vi "THzTimeScan_830_VC.vi"(0 "input":T1) -> (1 "loop stop":bool, 2 "x-axis":sgl[](array[numeric]), 3 "y-axis":dbl[](array[numeric]))   [LabVIEW 2010]
uses:
  <vilib>/Utility/file.llb/Write To Spreadsheet File (string).vi
panel:
  out "Position":dbl[](array[numeric])=[3.9963] format="%.6f"
  out "Array":dbl[](array[numeric])
  out "String":string
  out "Move delay":bool
  out "Read830":bool
  out "THz Signal Graph":dbl(graph)
  in  "loop stop":bool
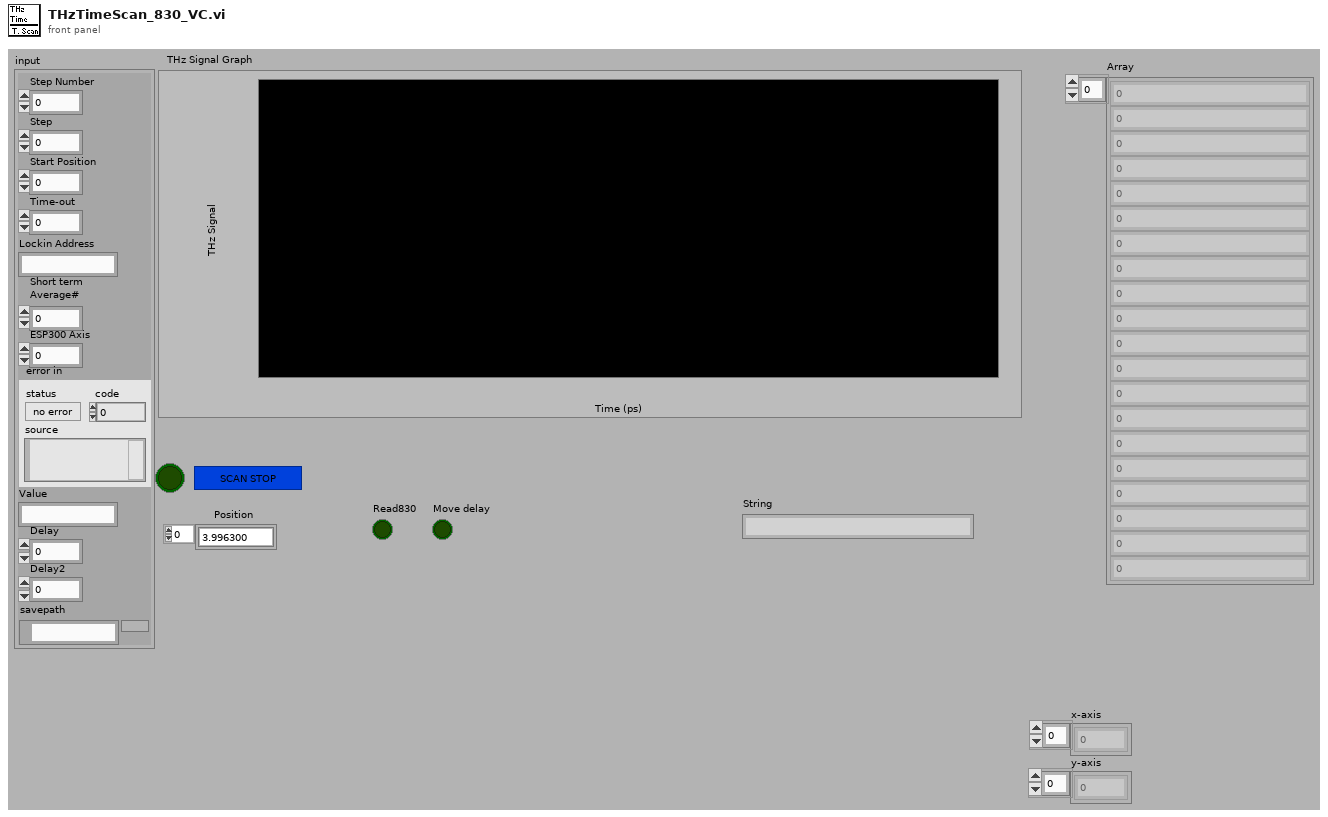
[diagram p1: front panel]
types:
  T1 = cluster{"Step Number":i32, "Step":sgl, "Start Position":sgl, "Time-out":i32, "Lockin Address":string, "Short term \nAverage#":i8, "ESP300 Axis":i8, "error in":errorcluster, "Value":string, "Delay":dbl, "Delay2":dbl, "savepath":path}
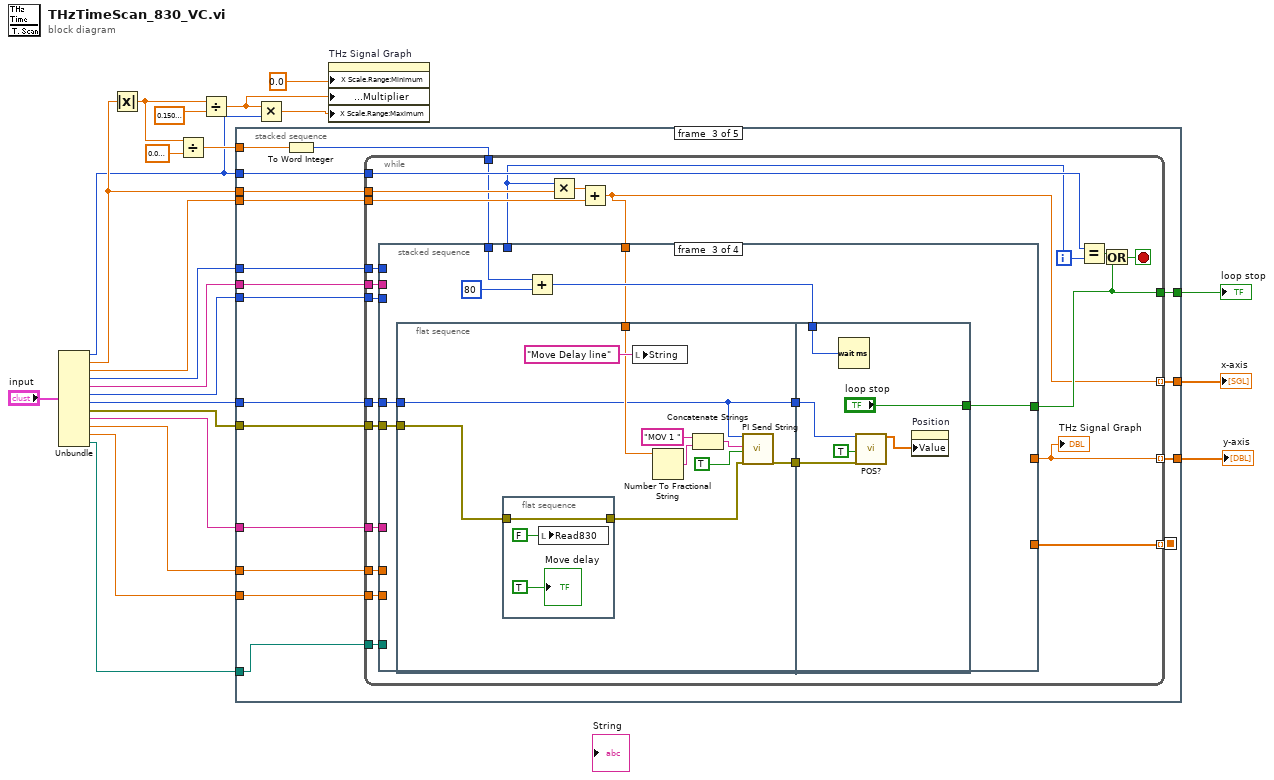
[diagram p0: block diagram]
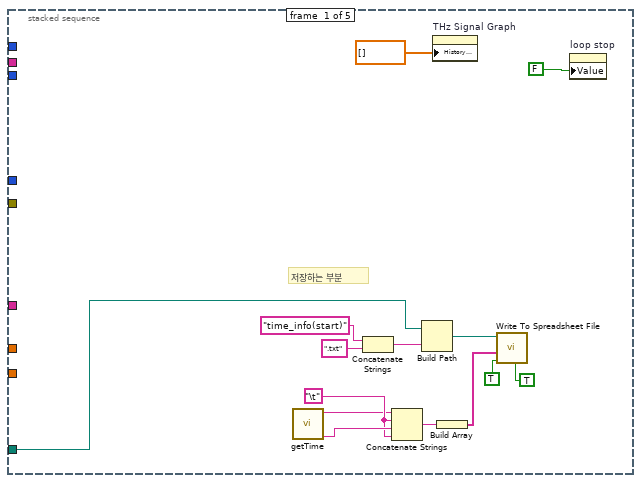
[diagram p2: hidden frame]
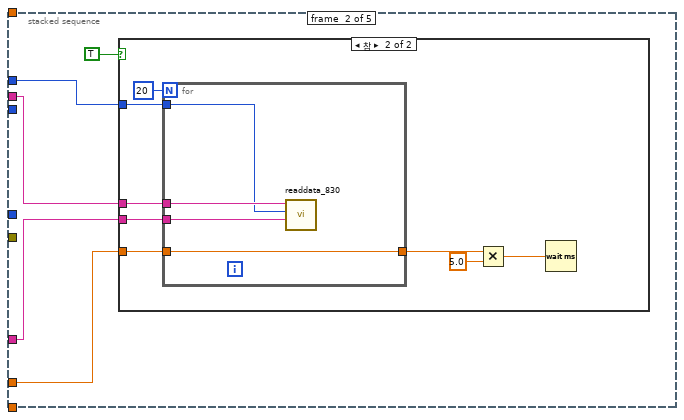
[diagram p3: hidden frame]
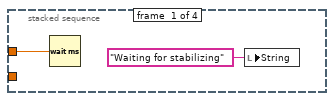
[diagram p5: hidden frame]
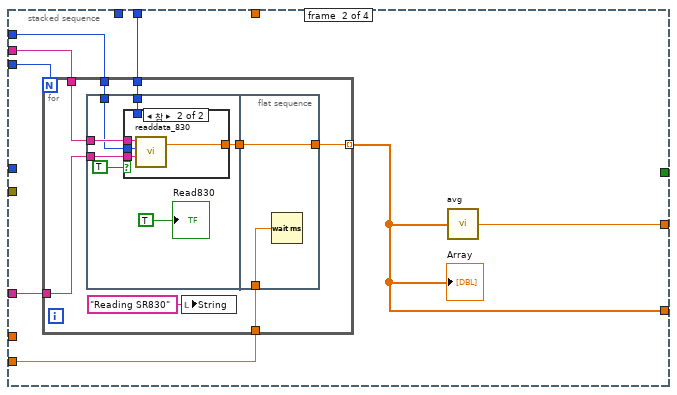
[diagram p6: hidden frame]
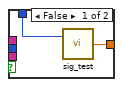
[diagram p7: hidden frame]
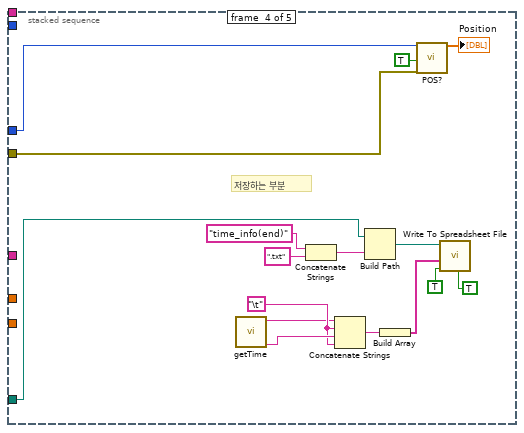
[diagram p9: hidden frame]
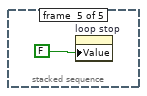
[diagram p10: hidden frame]
diagram:
  n1 = Unbundle("input") -> ("Step Number"=w9:i32, "Step"=w15:sgl, "Start Position"=w14:sgl, "Time-out"=w13:i32, "Lockin Address"=w12:string, "Short term \nAverage#"=w5:i8, "ESP300 Axis"=w11:i8, "error in"=w1:errorcluster, "Value"=w10:string, "Delay"=w4:dbl, "Delay2"=w3:dbl, "savepath"=w2:path)
  n2 = Absolute Value(x=w15) -> (abs(x)=w19:sgl)
  n3 = Divide(x=w19, y=sgl 0.004) -> (x/y=w17:sgl)
  n4 = Divide(x=w19, y=sgl 0.15) -> (x/y=w7:sgl)
  n5 = stacked-sequence {
    seq-local: [_ _ w58 _ _] -> [_ _ _ _ _]
    tunnel: w14 -> [_ _ w72 _ _]
    tunnel: w13 -> [_ w42 w71 _ _]
    tunnel: w12 -> [_ w41 w70 _ _]
    tunnel: w5 -> [_ _ w69 _ _]
    tunnel: w11 -> [_ _ w56 w156 _]
    tunnel: w1 -> [_ _ w55 w155 _]
    tunnel: w10 -> [_ w40 w61 _ _]
    tunnel: [_ _ w68 _ _] -> w23
    tunnel: [_ _ w67 _ _] -> w22
    tunnel: [_ _ w66 _ _] -> w21
    tunnel: w15 -> [_ _ w64 _ _]
    tunnel: w9 -> [_ _ w65 _ _]
    tunnel: w17 -> [_ _ w63 _ _]
    tunnel: w4 -> [_ w38 w60 _ _]
    tunnel: w3 -> [_ _ w59 _ _]
    tunnel: w2 -> [w24 _ w57 w159 _]
    frame #0 {
      w27 = "\t"
      # "저장하는 부분"
      n6 = call "getTime.vi"() -> ("시간"=w28:string, "날짜"=w26:string)  [unwired: 10 in]
      n7 = Concatenate Strings("time_info(start)" ("string"), ".txt" ("string")) -> (w34:string)
      n8 = Concatenate Strings(w26, w27, w28, w27) -> (w25:string)
      n9 = Build Path(base path=w24, name or relative path=w34) -> (appended path=w31:path)
      n10 = property on="THz Signal Graph" class="WFChart (엄격한)"("History Data"=dbl[] []) -> ()  [unwired: 2 in, 2 out]
      n11 = Build Array(w25) -> (w30:string[])
      n12 = call-poly <vilib>:"Write To Spreadsheet File.vi"("transpose? (no:F)"=TRUE ("transpose?\n(no:F)"), "append to file? (new file:F)"=TRUE ("transpose?\n(no:F)"), "1D data"=w30, "file path (dialog if empty)"=w31) -> ()  [unwired: 4 in, 1 out]
      n13 = property on="loop stop" class="Bool (엄격한)"("Value"=FALSE) -> ()  [unwired: 2 in, 2 out]
    }
    frame #1 {
      n14 = case shown="참" TRUE {
        tunnel: w42 -> [_ w49]
        tunnel: w41 -> [_ w48]
        tunnel: w40 -> [_ w47]
        tunnel: w38 -> [_ w46]
        frame False {
        }
        frame True {
          n15 = for {
            N: 20 -> [_]
            tunnel: w48 -> [w54]
            tunnel: w47 -> [w53]
            tunnel: w49 -> [w52]
            tunnel: w46 -> [w51]
            tunnel: [w51] -> w45
            n16 = call "readdata_830.vi"("Command"=w53, "timeout"=w52, "Lockin Address"=w54) -> ()  [unwired: 1 in, 2 out]
          }
          n17 = Multiply(x=w45, y=5.0) -> (x*y=w43:dbl)
          n18 = Wait (ms)(milliseconds to wait=w43) -> ()  [unwired: 1 out]
        }
      }
    }
    frame #2 {
      n19 = To Word Integer(number=w63) -> (16bit integer=w62:i16)
      n20 = while {
        tunnel: [w81] -> w68
        tunnel: [w85] -> w66 mode=indexing
        tunnel: [w75] -> w67 mode=indexing
        tunnel: w65 -> [w90]
        tunnel: w64 -> [w89]
        tunnel: w72 -> [w88]
        tunnel: w71 -> [w82]
        tunnel: w70 -> [w87]
        tunnel: w69 -> [w86]
        tunnel: w62 -> [w84]
        tunnel: w61 -> [w83]
        tunnel: w60 -> [w80]
        tunnel: w59 -> [w79]
        tunnel: [w78] -> w58 mode=indexing
        tunnel: w57 -> [w76]
        tunnel: w56 -> [w74]
        tunnel: w55 -> [w73]
        i -> [w77]
        stop <- w93 stop-if-true
        n21 = Multiply(x=w77, y=w89) -> (x*y=w91:sgl)
        n22 = Add(x=w91, y=w88) -> (x+y=w75:sgl)
        n23 = stacked-sequence {
          tunnel: w87 -> [_ w100 _ _]
          tunnel: [_ w102 _ _] -> w85
          tunnel: w86 -> [_ w103 _ _]
          tunnel: w84 -> [_ _ w135 _]
          tunnel: w83 -> [_ w101 _ _]
          tunnel: w82 -> [_ w99 _ _]
          tunnel: [_ _ w132 _] -> w81
          tunnel: w80 -> [w95 _ _ _]
          tunnel: w79 -> [_ w98 _ _]
          tunnel: [_ w97 _ _] -> w78
          tunnel: w77 -> [_ w96 _ _]
          tunnel: w76 -> [_ _ _ _]
          tunnel: w75 -> [_ _ w131 _]
          tunnel: w74 -> [_ _ w130 _]
          tunnel: w73 -> [_ _ w129 _]
          frame #0 {
            n24 = Wait (ms)(milliseconds to wait=w95) -> ()  [unwired: 1 out]
            n25 = local write "String"("Waiting for stabilizing" ("String")) -> ()
          }
          frame #1 {
            n26 = for {
              N: w103 -> [_]
              tunnel: w100 -> [w108]
              tunnel: w99 -> [w111]
              tunnel: [w110] -> w97 mode=indexing
              tunnel: w101 -> [w109]
              tunnel: w98 -> [w105]
              tunnel: w96 -> [w104]
              n27 = flat-sequence {
                tunnel: w111 -> [w115]
                tunnel: w109 -> [w116]
                tunnel: w108 -> [w117]
                tunnel: [w114] -> w106
                tunnel: w104 -> [w112]
                tunnel: [w126] -> w110
                tunnel: w106 -> [w126]
                tunnel: w105 -> [w125]
                frame #0 {
                  n28 = case shown="참" TRUE {
                    tunnel: w117 -> [_ w124]
                    tunnel: w116 -> [_ w123]
                    tunnel: w115 -> [_ w122]
                    tunnel: [w120 w121] -> w114
                    tunnel: w112 -> [w119 _]
                    frame False {
                      n29 = call "sig_test.vi"("index (row)"=w119) -> ("element"=w120:dbl)  [unwired: 1 in]
                    }
                    frame True {
                      n30 = call "readdata_830.vi"("Command"=w123, "timeout"=w122, "Lockin Address"=w124) -> ("Data"=w121:dbl)  [unwired: 1 in, 1 out]
                    }
                  }
                  "Read830" <- TRUE ("Read830")
                }
                frame #1 {
                  n31 = Wait (ms)(milliseconds to wait=w125) -> ()  [unwired: 1 out]
                }
              }
              n32 = local write "String"("Reading SR830" ("String")) -> ()
            }
            "Array" <- w97
            n33 = call "avg.vi"("Array"=w97) -> ("Numeric"=w102:dbl)
          }
          frame #2 {
            n34 = flat-sequence {
              tunnel: w131 -> [w140]
              tunnel: w130 -> [w136]
              tunnel: w129 -> [w139]
              tunnel: [w137] -> w128
              tunnel: [w136] -> w127
              tunnel: w134 -> [w153]
              tunnel: ["loop stop"] -> w132
              tunnel: w128 -> [w151]
              tunnel: w127 -> [w150]
              frame #0 {
                n35 = flat-sequence {
                  tunnel: [w148] -> w138
                  tunnel: w139 -> [w148]
                  frame #0 {
                    n36 = local write "Read830"(FALSE ("Read830")) -> ()
                    "Move delay" <- TRUE ("Move delay")
                  }
                }
                n37 = local write "String"("Move Delay line" ("String")) -> ()
                n38 = Number To Fractional String(number=w140) -> (F-format string=w144:string)  [unwired: 3 in]
                n39 = Concatenate Strings("MOV 1 ", w144) -> (w141:string)
                n40 = call "PI Send String.vi"("System no."=w136, "String to send"=w141, "Attach termination char.?"=TRUE ("Attach Linefeed?"), "error in"=w138) -> ("error out"=w137:errorcluster)  [unwired: 15 in]
              }
              frame #1 {
                n41 = Wait (ms)(milliseconds to wait=w153) -> ()  [unwired: 1 out]
                n42 = call "POS?.vi"("System no."=w150, "All axes?"=TRUE, "error in"=w151) -> ("Position"=w149:dbl[])  [unwired: 15 in, 1 out]
                n43 = property on="Position" class="Arr (엄격한)"("Value"=w149) -> ()  [unwired: 2 in, 2 out]
              }
            }
            n44 = Add(x=w135, y=i16 80) -> (x+y=w134:i16)
          }
          frame #3 {
          }
        }
        "THz Signal Graph" <- w85
        n45 = Equal?(x=w90, y=w77) -> (x = y?=w92:bool)
        n46 = Or(x=w92, y=w81) -> (x .or. y?=w93:bool)
      }
    }
    frame #3 {
      w162 = "\t"
      # "저장하는 부분"
      n47 = call "getTime.vi"() -> ("시간"=w163:string, "날짜"=w161:string)  [unwired: 10 in]
      n48 = Concatenate Strings("time_info(end)" ("string"), ".txt" ("string")) -> (w169:string)
      n49 = Concatenate Strings(w161, w162, w163, w162) -> (w160:string)
      n50 = Build Path(base path=w159, name or relative path=w169) -> (appended path=w166:path)
      n51 = Build Array(w160) -> (w165:string[])
      n52 = call "POS?.vi"("System no."=w156, "All axes?"=TRUE, "error in"=w155) -> ("Position"=→"Position":dbl[])  [unwired: 15 in, 1 out]
      n53 = call-poly <vilib>:"Write To Spreadsheet File.vi"("transpose? (no:F)"=TRUE ("transpose?\n(no:F)"), "append to file? (new file:F)"=TRUE ("transpose?\n(no:F)"), "1D data"=w165, "file path (dialog if empty)"=w166) -> ()  [unwired: 4 in, 1 out]
    }
    frame #4 {
      n54 = property on="loop stop" class="Bool (엄격한)"("Value"=FALSE) -> ()  [unwired: 2 in, 2 out]
    }
  }
  "loop stop" <- w23
  "x-axis" <- w22
  "y-axis" <- w21
  n55 = Multiply(x=w7, y=w9) -> (x*y=w6:sgl)
  n56 = property on="THz Signal Graph" class="WFChart (엄격한)"("X Scale.Range:Minimum"=0.0, "X Scale.Offset and Multiplier:Multiplier"=w7, "X Scale.Range:Maximum"=w6) -> ()  [unwired: 2 in, 2 out]
